vi "Check for Valid Lock Out Hash.vi"(8 "error in":errorcluster, 10 "Key In":string, 11 "Refnum in":T2) -> (0 "error out":errorcluster, 1 "Sorted Data":T1, 2 "HashGood?":bool, 3 "Refnum out":T2)   [LabVIEW 2013]
uses:
  <vilib>/Utility/config.llb/Config Data RefNum.ctl
  <userlib>/_OpenG.lib/array/array.llb/Sort 1D Array (DBL)__ogtk.vi
  <vilib>/Utility/config.llb/Read Key (Double).vi
  <vilib>/Utility/config.llb/Read Key (String).vi
  <vilib>/Utility/config.llb/NI_LVConfig.lvlib
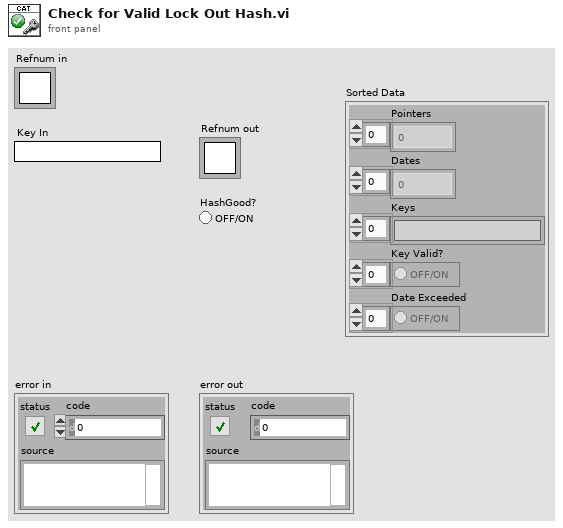
[diagram p1: front panel]
types:
  T1 = cluster{"Pointers":i32[], "Dates":dbl[], "Keys":string[], "Key Valid?":bool[], "Date Exceeded":bool[]}
  T2 = typedef "NI_LVConfig.lvlib/Config Data RefNum.ctl" = refnum<k1>
  T3 = cluster{"Pointers":i32[], "Dates":dbl[], "Keys":string[], "Key Valid?":bool[], "Key Valid? 2":bool[]}
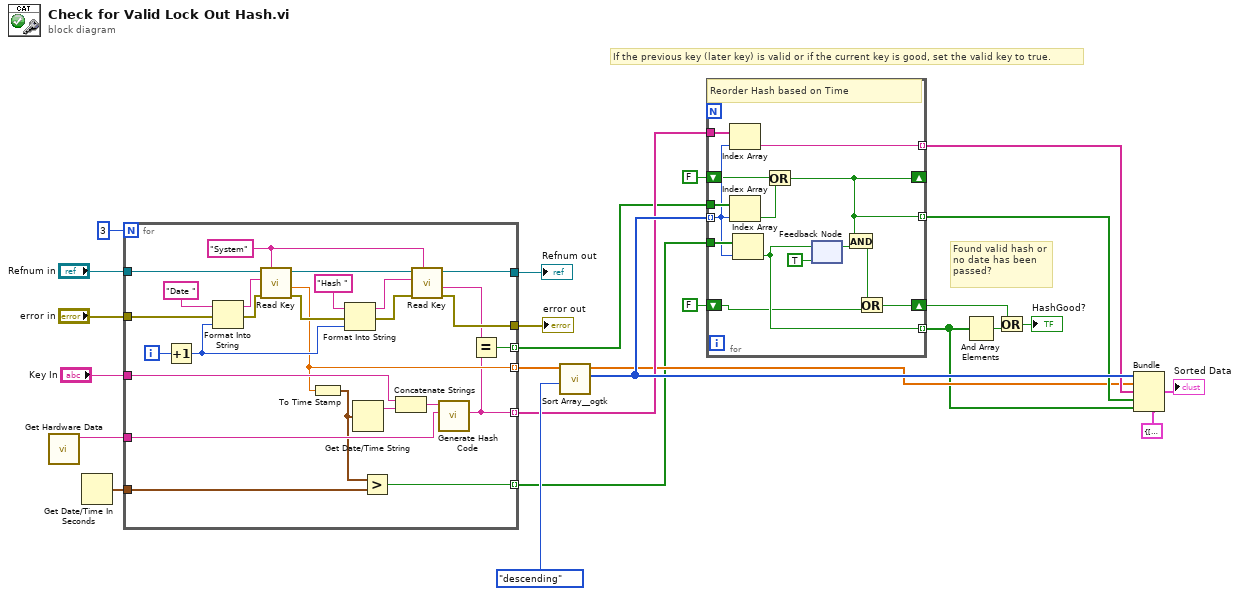
[diagram p0: block diagram]
diagram:
  # "If the previous key (later key) is valid or if the current key is good, set the valid key to true."
  # "Found valid hash or no date has been passed?"
  n1 = call "Get Hardware Data.vi"() -> ("Fingerprint"=w14:string)  [unwired: 11 in]
  n2 = Get Date/Time In Seconds() -> (seconds since 1Jan1904=w6:timestamp)
  n3 = for {
    N: 3 -> [_]
    tunnel: "Refnum in" -> [w43]
    tunnel: [w32] -> w22 mode=indexing
    tunnel: [w42] -> w16
    tunnel: [w41] -> w15
    tunnel: "error in" -> [w40]
    tunnel: w14 -> [w34]
    tunnel: "Key In" -> [w33]
    tunnel: [w30] -> w10 mode=indexing
    tunnel: [w29] -> w12 mode=indexing
    tunnel: w6 -> [w28]
    tunnel: [w26] -> w5 mode=indexing
    i -> [w39]
    w37 = "System" ("section")
    n4 = Increment(x=w39) -> (x+1=w38:i32)
    n5 = Format Into String(initial string="Date " ("key"), error in=w40, w38) -> (resulting string=w49:string, error out=w48:errorcluster)  [unwired: 1 in]
    n6 = call-poly <vilib>:"Read Key.vi"("section"=w37, "error in (no error)"=w48, "key"=w49, "refnum"=w43) -> ("error out"=w47:errorcluster, "value"=w32:dbl, "refnum out"=w51:T2)  [unwired: 4 in, 1 out]
    n7 = To Time Stamp(1:w32) -> (0:w27:timestamp)
    n8 = Format Into String(initial string="Hash " ("key"), error in=w47, w38) -> (resulting string=w50:string, error out=w46:errorcluster)  [unwired: 1 in]
    n9 = Get Date/Time String(seconds (now)=w27) -> (date string=w36:string)  [unwired: 2 in, 1 out]
    n10 = Greater?(x=w27, y=w28) -> (0:w26:bool)
    n11 = Concatenate Strings(w33, w36) -> (w35:string)
    n12 = call-poly <vilib>:"Read Key.vi"("section"=w37, "error in (no error)"=w46, "key"=w50, "refnum"=w51) -> ("error out"=w41:errorcluster, "value"=w31:string, "refnum out"=w42:T2)  [unwired: 4 in, 1 out]
    n13 = call "Generate Hash Code.vi"("Fingerprint"=w34, "Product ID"=w35) -> ("Hash"=w29:string)  [unwired: 8 in, 1 out]
    n14 = Equal?(x=w31, y=w29) -> (x = y?=w30:bool)
  }
  "error out" <- w15
  "Refnum out" <- w16
  n15 = call-poly <userlib>:"Sort Array__ogtk.vi"("Order"=enum16{"ascending", "descending"}."descending", "Array in"=w22) -> ("Sorted Pointers"=w20:i32[], "Sorted Array out"=w7:dbl[])  [unwired: 8 in]
  n16 = for {
    tunnel: w20 -> [w61] mode=indexing
    tunnel: w12 -> [w65]
    tunnel: w10 -> [w63]
    tunnel: [w64] -> w11 mode=indexing
    tunnel: [w53] -> w8 mode=indexing
    tunnel: w5 -> [w62]
    tunnel: [w58] -> w1 mode=indexing
    shift-right: [w56] -> w3
    shift-left: FALSE -> [w55]
    shift-right: [w53] -> _
    shift-left: FALSE -> [w52]
    # "Reorder Hash based on Time"
    n17 = Index Array(array=w65, index=w61) -> (element=w64:string)
    n18 = Index Array(array=w63, index=w61) -> (element=w54:bool)
    n19 = Index Array(array=w62, index=w61) -> (element=w58:bool)
    n20 = Or(x=w52, y=w54) -> (x .or. y?=w53:bool)
    n21 = feedback #1(TRUE) -> (w59:bool)
    n22 = feedback-in #1(w58) -> ()
    n23 = And(x=w53, y=w59) -> (x .and. y?=w57:bool)
    n24 = Or(x=w57, y=w55) -> (x .or. y?=w56:bool)
  }
  n25 = And Array Elements(Boolean array=w1) -> (logical AND=w24:bool)
  n26 = Or(x=w3, y=w24) -> (x .or. y?=→"HashGood?":bool)
  n27 = Bundle(cluster=T3 {"Pointers"=[], "Dates"=[], "Keys"=[], "Key Valid?"=[], "Key Valid? 2"=[]} ("Sorted Data"), "Pointers"=w20, "Dates"=w7, "Keys"=w11, "Key Valid?"=w8, "Key Valid? 2"=w1) -> (→"Sorted Data":T3)
